vi "Test_5782_DC_level.vi"() -> ()   [LabVIEW 2013]
uses:
  <vilib>/userdefined/High Color/nirio_resource_hc.ctl
  <vilib>/Analysis/baseanly.llb/Mean (DBL).vi
  <vilib>/FPGAPlugInAG/PXIe-7975R/niLvFpga_Open_PXIe-7975R.vi
  <vilib>/rvi/interface/common/dynamic/niFpgaDynamicAddResources.vi
  <vilib>/rvi/interface/common/niFpgaWaitOnOcc.vi
  <vilib>/Utility/error.llb/Error Cluster From Error Code.vi
  <vilib>/rvi/errors/niLvFpgaAdjustHostInterfaceError.vi
  <vilib>/rvi/interface/nirviOpenFPGA/nirviOpenFPGA.xnode
  FPGA Bitfiles/mixer_FPGATarget2_5782inputtest_r0B46DafvIs.lvbitx
  <vilib>/rvi/interface/nirviMethod/nirviMethod.xnode
  <vilib>/rvi/interface/nirviReadWriteControl/nirviReadWriteControl.xnode
  <vilib>/rvi/errors/niLvFpgaMergeErrorWithErrorCode.vi
  <vilib>/FPGAPlugInAG/Dynamic/niLvFpga_ReadFifo_Dynamic.vi
  NiFpgaLv.dll
  <vilib>/rvi/interface/Simulation/niFpgaSimulationCallBeginRW.vi
  <vilib>/FPGAPlugInAG/Dynamic/niLvFpga_ConfigureFifo_Dynamic.vi
  <vilib>/FPGAPlugInAG/Dynamic/niLvFpga_StartFifo_Dynamic.vi
  <vilib>/Analysis/NI_AALBase.lvlib
panel:
  out "mean 2":dbl format="%0.2f"
  in  "mean":bool
  out "Waveform Chart":i16[][](graph)
  in  "stop":bool
  in  "Downsample rate":u32=500
  in  "Measure":bool
  in  "resource name":T1="RIO0"
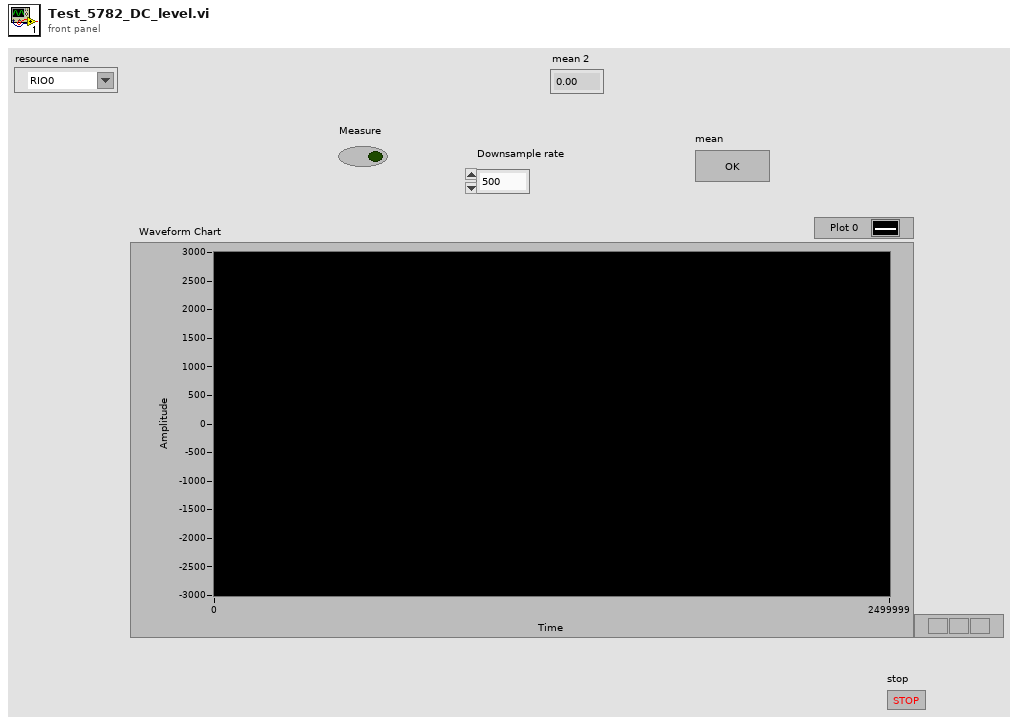
[diagram p1: front panel]
types:
  T1 = typedef "nirio_resource_hc.ctl" = tag
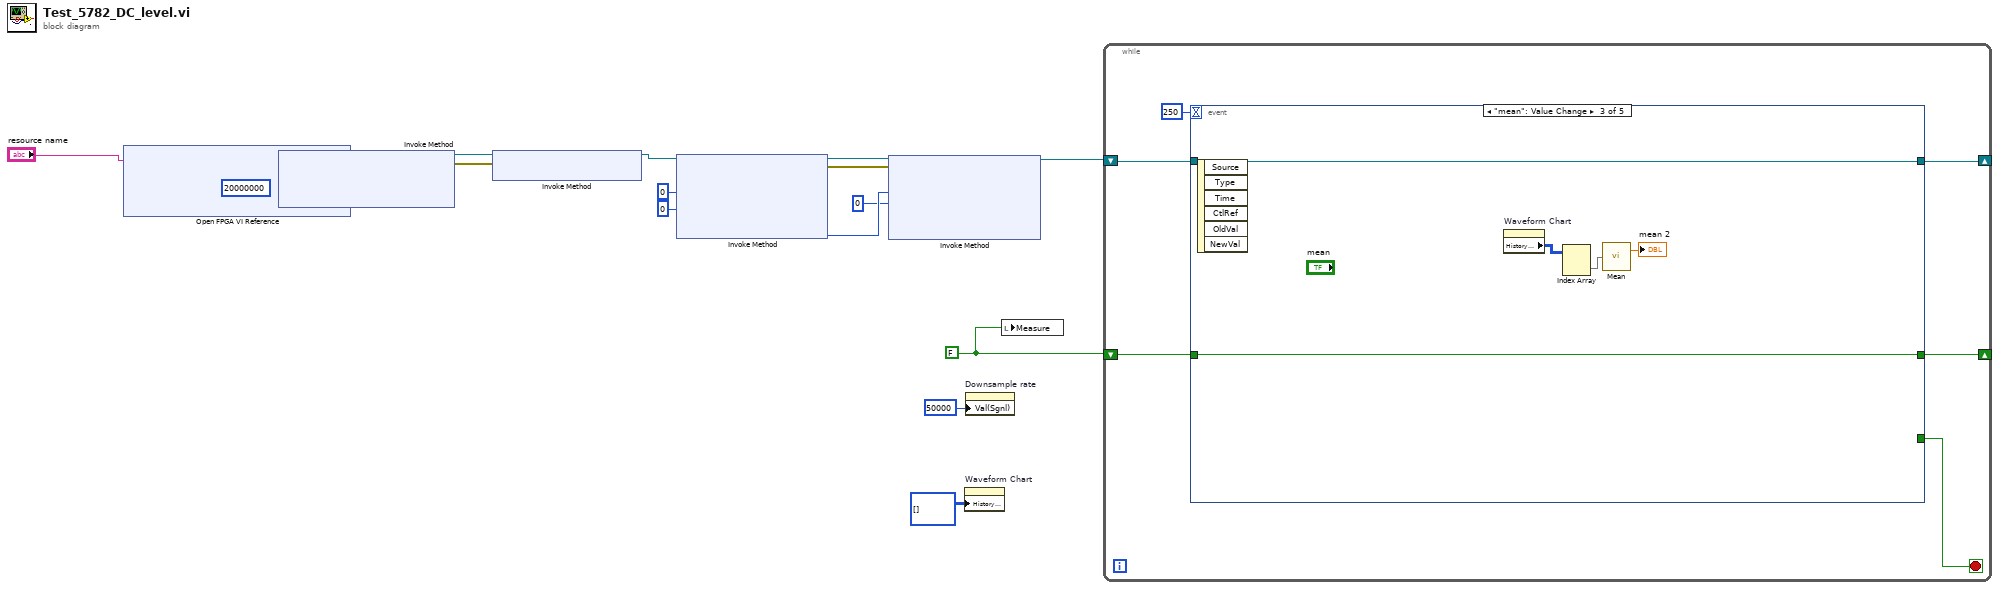
[diagram p0: block diagram]
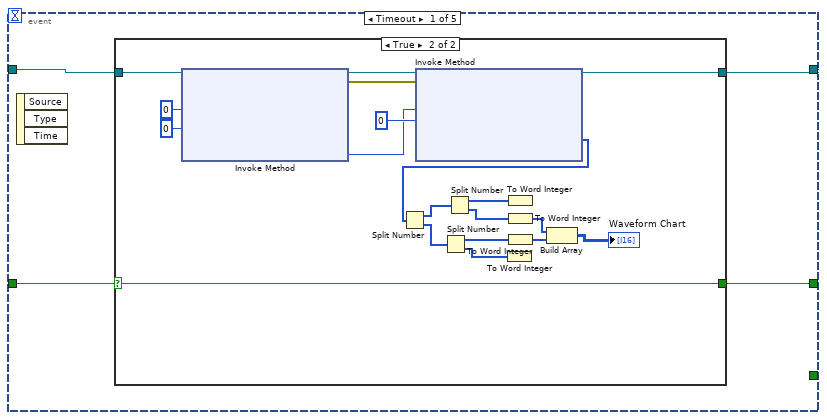
[diagram p2: hidden frame]
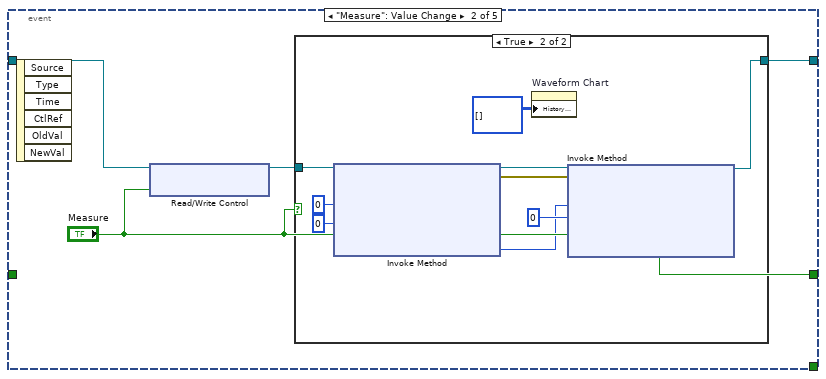
[diagram p4: hidden frame]
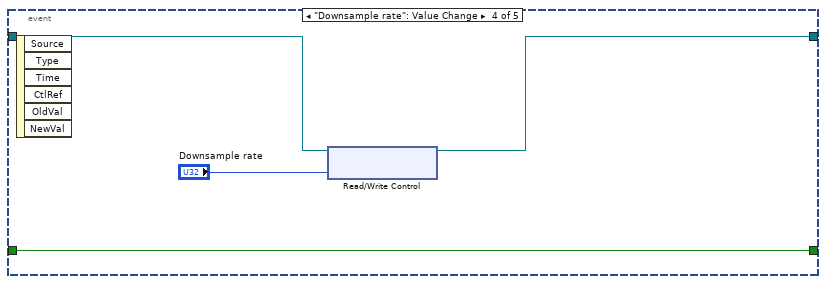
[diagram p6: hidden frame]
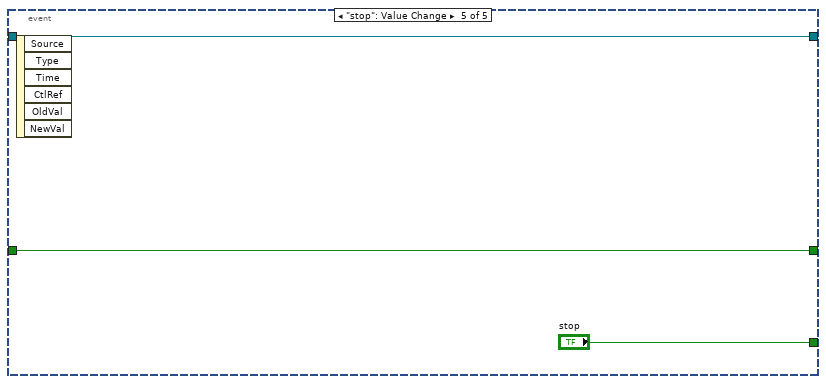
[diagram p7: hidden frame]
diagram:
  w2 = FALSE ("Measure")
  n1 = xnode "Open FPGA VI Reference"("resource name"="resource name") -> ("FPGA VI Reference Out"=w6:refnum<k20>)  [unwired: 1 in, 1 out]
  n2 = xnode "Invoke Method"("FPGA VI Reference In"=w6, "Requested Depth"=u32 20000000 ("Depth")) -> ("FPGA VI Reference Out"=w13:refnum<k20>, "error out"=w14:errorcluster)  [unwired: 1 in, 1 out]
  n3 = xnode "Invoke Method"("FPGA VI Reference In"=w13, "error in"=w14) -> ("FPGA VI Reference Out"=w5:refnum<k20>)  [unwired: 1 out]
  n4 = xnode "Invoke Method"("FPGA VI Reference In"=w5, "Number of Elements"=u32 0, "Timeout (ms)"=0) -> ("FPGA VI Reference Out"=w8:refnum<k20>, "error out"=w7:errorcluster, "Elements Remaining"=w10:u32)  [unwired: 1 in, 1 out]
  n5 = xnode "Invoke Method"("FPGA VI Reference In"=w8, "error in"=w7, "Number of Elements"=w10, "Timeout (ms)"=0) -> ("FPGA VI Reference Out"=w4:refnum<k20>)  [unwired: 3 out]
  n6 = property on="Waveform Chart" class="WFChart (strict)"("History Data"=i16[][] []) -> ()  [unwired: 2 in, 2 out]
  n7 = property on="Downsample rate" class="DigNum (strict)"("Val(Sgnl)"=u32 50000 ("Value (Signaling)")) -> ()  [unwired: 2 in, 2 out]
  n8 = local write "Measure"(w2) -> ()
  n9 = while {
    shift-right: [w19] -> _
    shift-left: w2 -> [w20]
    shift-right: [w17] -> _
    shift-left: w4 -> [w22]
    stop <- w18 stop-if-true
    n10 = event shown="[2] \"mean\": Value Change" {
      selector: _ -> [_ _ _ _ _]
      dyn-events: _ -> [_ _ _ _ _]
      timeout: 250 -> [_ _ _ _ _]
      tunnel: w22 -> [w26 w51 w65 w68 w71]
      tunnel: w20 -> [w25 _ w66 w69 w72]
      tunnel: [w24 "Measure" w66 w69 w72] -> w19
      tunnel: [_ _ _ _ "stop"] -> w18
      tunnel: [w23 w48 w65 w67 w71] -> w17
      event Timeout {
        n11 = event-data() -> ()  [unwired: 1 in, 3 out]
        n12 = case shown="True" w25 {
          selector: w25 -> [w28 w33]
          tunnel: w26 -> [w27 w41]
          tunnel: [w28 w33] -> w24
          tunnel: [w27 w32] -> w23
          frame False {
          }
          frame True {
            n13 = xnode "Invoke Method"("FPGA VI Reference In"=w41, "Number of Elements"=u32 0, "Timeout (ms)"=0) -> ("FPGA VI Reference Out"=w46:refnum<k20>, "error out"=w47:errorcluster, "Elements Remaining"=w44:u32)  [unwired: 1 in, 1 out]
            n14 = xnode "Invoke Method"("FPGA VI Reference In"=w46, "error in"=w47, "Number of Elements"=w44, "Timeout (ms)"=0) -> ("FPGA VI Reference Out"=w32:refnum<k20>, "Data"=w34:u64[])  [unwired: 2 out]
            n15 = Split Number(x=w34) -> (hi(x)=w39:u32[], lo(x)=w35:u32[])
            n16 = Split Number(x=w35) -> (hi(x)=w37:u16[], lo(x)=w38:u16[])
            n17 = Split Number(x=w39) -> (hi(x)=w40:u16[], lo(x)=w36:u16[])
            n18 = To Word Integer(number=w38) -> ()  [unwired: 1 out]
            n19 = To Word Integer(number=w40) -> ()  [unwired: 1 out]
            n20 = To Word Integer(number=w36) -> (16bit integer=w31:i16[])
            n21 = To Word Integer(number=w37) -> (16bit integer=w30:i16[])
            n22 = Build Array(w31, w30) -> (→"Waveform Chart":i16[][])
          }
        }
      }
      event "Measure": Value Change {
        n23 = event-data() -> ()  [unwired: 1 in, 6 out]
        n24 = xnode "Read/Write Control"("FPGA VI Reference In"=w51, "Trigger Acquisition"="Measure") -> ("FPGA VI Reference Out"=w49:refnum<k20>)  [unwired: 1 in, 1 out]
        n25 = case shown="True" "Measure" {
          tunnel: w49 -> [w52 w55]
          tunnel: [w52 w54] -> w48
          frame False {
          }
          frame True {
            n26 = xnode "Invoke Method"("FPGA VI Reference In"=w55, "Number of Elements"=u32 0, "Timeout (ms)"=0) -> ("FPGA VI Reference Out"=w60:refnum<k20>, "error out"=w61:errorcluster, "Elements Remaining"=w58:u32)  [unwired: 1 in, 1 out]
            n27 = property on="Waveform Chart" class="WFChart (strict)"("History Data"=i16[][] []) -> ()  [unwired: 2 in, 2 out]
            n28 = xnode "Invoke Method"("FPGA VI Reference In"=w60, "error in"=w61, "Number of Elements"=w58, "Timeout (ms)"=0) -> ("FPGA VI Reference Out"=w54:refnum<k20>)  [unwired: 3 out]
          }
        }
      }
      event "mean": Value Change {
        n29 = event-data() -> ()  [unwired: 1 in, 6 out]
        n30 = property on="Waveform Chart" class="WFChart (strict)"() -> ("History Data"=w64:i16[][])  [unwired: 2 in, 2 out]
        n31 = Index Array(array=w64) -> (element=w63:i16[])  [unwired: 2 in]
        n32 = call-poly <vilib>:"Mean.vi"("X"=w63) -> ("mean"=→"mean 2":dbl)  [unwired: 1 out]
      }
      event "Downsample rate": Value Change {
        n33 = event-data() -> ()  [unwired: 1 in, 6 out]
        n34 = xnode "Read/Write Control"("FPGA VI Reference In"=w68, "downsample rate"="Downsample rate") -> ("FPGA VI Reference Out"=w67:refnum<k20>)  [unwired: 1 in, 1 out]
      }
      event "stop": Value Change {
        n35 = event-data() -> ()  [unwired: 1 in, 6 out]
      }
    }
  }
